vi "AlliGator Compute Optimal IRF v2.vi"(0 "Selected Plot Info":T8={"Multiplot XY Graph"=refnum, "Mouse Coordinates"={"Horizontal"=0, "Vertical"=0}, "Plot Index"=-1}, 5 "IRF*PSED Fixed Parameters":T3={"order"=0, "T"=0.0, "Time Constant Array"=[], "{S_k, C_k, phi_k, e_k} arrays"={"S_k Array"=[], "C_k Array"=[], "phi_k Array"=[], "e_k Array"=[]}, "IRF Extraction Options"={"Time Constant for IRF Extraction"=1e-18, "IRF Order"=0, "Fourier Series Smoothing"=enum."None", "Noise Threshold"=0.0, "Smoothing Width"=0.0, "Fourier Series Truncation"=enum."Automatic", "Truncation Order"=0, "Save Power Spectrum"=FALSE, "Smoothing"=FALSE, "Smoothing Parameter"=0.0, "Smoothing Order"=1, "Method"=enum."Direct"}} {"IRF Extraction Options"."Smoothing Order" min=1 max=10; "IRF Extraction Options"."Time Constant for IRF Extraction" format="%#_5g"}, 9 "IRF Optimization Control":T1={"Search Range"=1e-18, "Search Step"=1e-18, "Tail Threshold (%)"=1e-09, "Regularized IRF"=FALSE, "Export Plot"=FALSE, "Export Data"=FALSE, "Smooth Metrics"=FALSE, "S-G Side Points"=1, "S-G Polynomial Order"=3, "Metrics"=enum."Average"} {"S-G Polynomial Order" min=3 max=10; "S-G Side Points" min=1; "Tail Threshold (%)" min=0.0 max=100.0; "Search Range" min=0.0 max=1e-09}, 11 "Error In":errorcluster) -> (2 "Optimization Graph":cluster{"Ramp Pattern":dbl[], dbl[]}[](graph), 3 "Residuals Plot":cluster{"X Array":dbl[], "Y Array":dbl[]}, 4 "Fitted Plot":cluster{"X Array":dbl[], "Y Array":dbl[]}, 6 "Plot Name":string, 8 "Fit Parameter Values":dbl[](array[numeric]), 10 "Optimal Tau":dbl, 13 "Additional Data":variant, 14 "Fit Results String":string, 15 "Error Out":errorcluster)   [LabVIEW 2021, in "AlliGator IRF.lvlib"]
doc: "Extract IRF from provided decay using deconvolution and finding the minimal metrics."
uses:
  AlliGator IRF.lvlib
  <vilib>/Analysis/NI_AALBase.lvlib
  Settings/AlliGator Settings.lvlib
  Settings/AlliGator Settings List.ctl
  Time/Time.lvlib
  Fits/Fit Calculation Method.ctl
  Fits/Fits.lvlib
  Fits/Residual Type.ctl
  Fits/Decay Convolution/Decay Model.ctl
  Fits/Ramp Type.ctl
  <vilib>/Analysis/6fits.llb/Curve Fitting Criteria.ctl
  <vilib>/Analysis/NI_AALPro.lvlib
  Fits/Fit Settings.ctl
  Fits/D-Only Fixed Parameters.ctl
  Fits/Fit Models.ctl
  Fits/IRF(X)PSED/IRF(X)PSED Fit Parameters.ctl
  <vilib>/Utility/miscctls.llb/LVPointDoubleTypeDef.ctl
  Fits/Fit Plot Request Information.ctl
  Error/Error.lvlib
  Fits/Non-linear Fitting Algorithm.ctl
  Utilities/Utilities.lvlib
  Fits/IRF(X)PSED/Fourier Series Smoothing Option.ctl
  Fits/IRF(X)PSED/Fourier Series Truncation.ctl
  Fits/IRF(X)PSED/IRF(X)PSED Extraction Options.ctl
  Fits/IRF(X)PSED/IRF Extraction Method.ctl
  Fits/Non-linear Fitting Method v2.ctl
  Fits/Nonlinear Fit Method.ctl
  <vilib>/Analysis/1siggen.llb/Ramp Pattern by Delta.vi
  Fits/IRF(X)PSED/Fit Weights Type v2.ctl
  Fits/IRF(X)PSED/Decay Fit Options v4.ctl
  <vilib>/Utility/miscctls.llb/LVPoint32TypeDef.ctl
  Graphs/XY Graph/XY Graph Refnum.ctl
  Graphs/XY Graph/XY Graph Add-Ons.lvlib
  Graphs/XY Graph/XY Graph Selected Plot Info.ctl
  Fits/IRF(X)PSED/IRF(X)PSED Fixed Parameters v3.ctl
  AlliGator IRF Optimization Controls.ctl
  AlliGator IRF Deconvolution Metrics.ctl
panel:
  in  "Minimum Type":enum16{"Integral", "Chi 2", "Product"}(ring)=enum."Chi 2"
  out "Current Tau (ns)":dbl format="%#_4g"
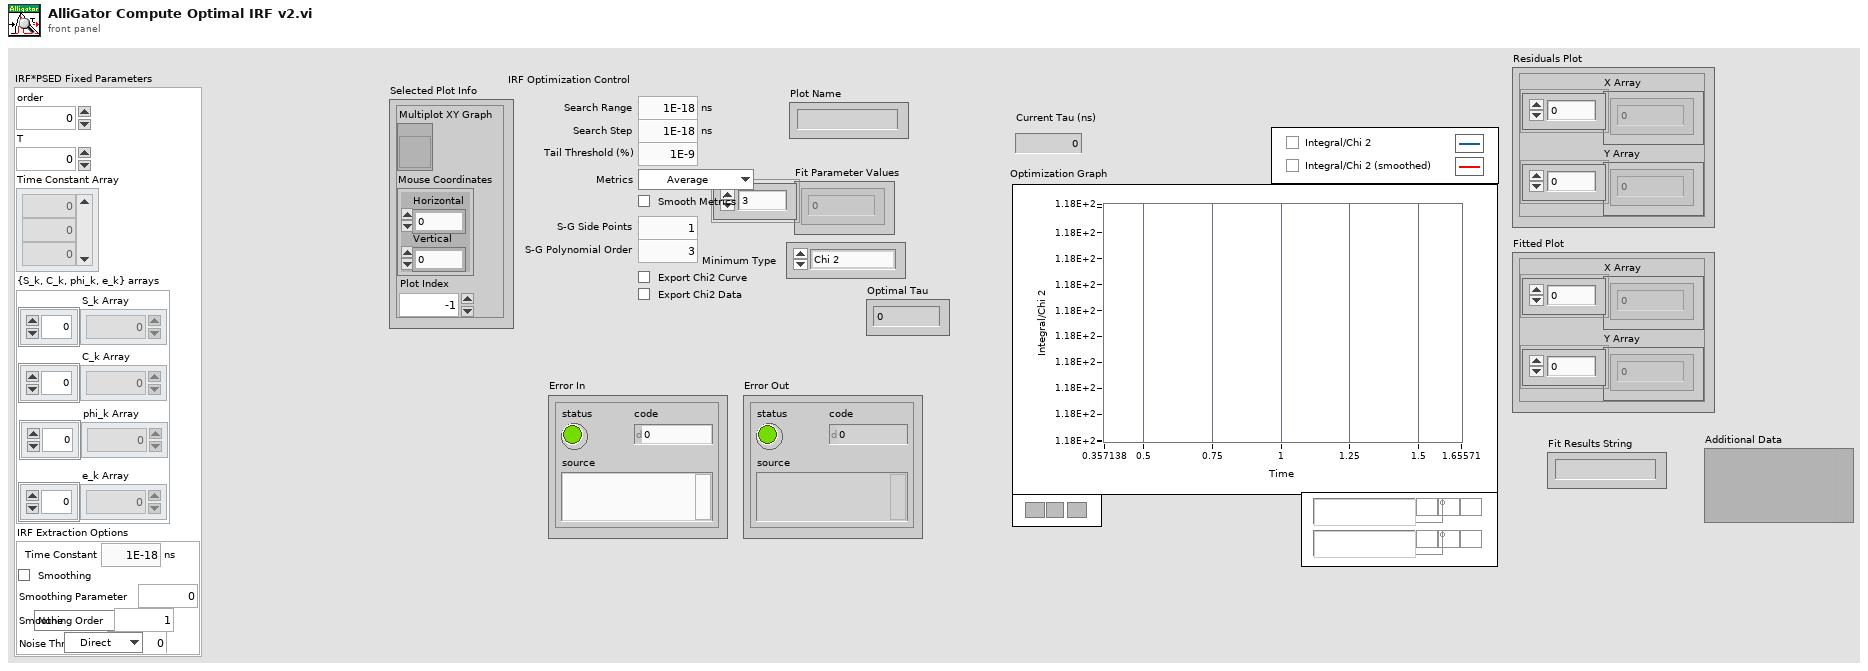
[diagram p1: front panel]
types:
  T1 = typedef "AlliGator IRF.lvlib/AlliGator IRF Optimization Controls.ctl" = cluster{"Search Range":dbl[unit], "Search Step":dbl[unit], "Tail Threshold (%)":dbl, "Regularized IRF":bool, "Export Plot":bool, "Export Data":bool, "Smooth Metrics":bool, "S-G Side Points":i32, "S-G Polynomial Order":i32, "Metrics":T2}
  T2 = typedef "AlliGator IRF.lvlib/AlliGator IRF Deconvolution Metrics.ctl" = enum16{"Average", "SDV", "Max", "Average * SDV", "Slope"}
  T3 = typedef "Fits.lvlib/IRF(X)PSED Fixed Parameters v3.ctl" = cluster{"order":i32, "T":dbl, "Time Constant Array":dbl[], "{S_k, C_k, phi_k, e_k} arrays":cluster{"S_k Array":dbl[], "C_k Array":dbl[], "phi_k Array":dbl[], "e_k Array":dbl[]}, "IRF Extraction Options":T4}
  T4 = typedef "Fits.lvlib/IRF(X)PSED Extraction Options.ctl" = cluster{"Time Constant for IRF Extraction":dbl[unit], "IRF Order":i32, "Fourier Series Smoothing":T5, "Noise Threshold":dbl, "Smoothing Width":dbl, "Fourier Series Truncation":T6, "Truncation Order":i32, "Save Power Spectrum":bool, "Smoothing":bool, "Smoothing Parameter":dbl, "Smoothing Order":u32, "Method":T7}
  T5 = typedef "Fits.lvlib/Fourier Series Smoothing Option.ctl" = enum16{"None", "Lanczos Factors", "Fejer Summation"}
  T6 = typedef "Fits.lvlib/Fourier Series Truncation.ctl" = enum16{"Automatic", "Fixed"}
  T7 = typedef "Fits.lvlib/IRF Extraction Method.ctl" = enum16{"Direct", "Topless", "Toeplitz"}
  T8 = typedef "XY Graph Add-Ons.lvlib/XY Graph Selected Plot Info.ctl" = cluster{"Multiplot XY Graph":T9, "Mouse Coordinates":T10, "Plot Index":i32}
  T9 = typedef "XY Graph Add-Ons.lvlib/XY Graph Refnum.ctl" = refnum<vi>
  T10 = typedef "LVPoint32TypeDef.ctl" = cluster{"Horizontal":i32, "Vertical":i32}
  T11 = typedef "Fits.lvlib/Fit Settings.ctl" = cluster{"Use Original Plot # Points":bool, "# Fit Plot Points":u32, "Fitting Method":T12, "Weighted Fit":T13, "Show All Fit Components":bool, "Axis Type":T14, "Show Fit Residuals":bool, "Residual Type":T15, "Fitting Algorithm":T16, "Show Confidence Interval":bool, "Confidence Level":dbl}
  T12 = typedef "Fits.lvlib/Nonlinear Fit Method.ctl" = enum16{"Least Square", "Least Absolute Residual", "Bisquare", "MLE"}
  T13 = typedef "Fits.lvlib/Fit Weights Type v2.ctl" = enum16{"Unweighted", "1/Variance (Neyman)", "1/Variance (Pearson)", "Best of All"}
  T14 = typedef "Fits.lvlib/Ramp Type.ctl" = u16
  T15 = typedef "Fits.lvlib/Residual Type.ctl" = enum16{"Standard", "Normalized", "Reduced"}
  T16 = typedef "Fits.lvlib/Non-linear Fitting Algorithm.ctl" = enum16{"Levenberg-Marquardt", "Trust-Region Dogleg"}
  T17 = typedef "Fits.lvlib/Decay Fit Options v4.ctl" = cluster{"Show Fit Residuals":bool, "Fit Model":T18, "Residual Type":T15, "Max Decay Percentile":dbl, "Min Decay Percentile":dbl, "Show Full Decay":bool, "Weights":T13, "Fitting Method":T19, "Compute Parameter Uncertainties":bool, "Periodic Boundaries":bool, "Model Calculation":T20, "Period":dbl[unit], "Termination Criteria":cluster{"Max Iterations":i32, "Max Function Calls":i32, "Max Time":dbl[unit], "Function Tolerance":dbl, "Parameter Tolerance":dbl, "Gradient Tolerance":dbl, "Min Lambda":dbl, "Max Lambda":dbl, "Initial Tick Count":u32}, "Offset Resolution":dbl[unit], "Use Local IRF":bool, "Fitting Algorithm":T16, "Show Confidence Interval ":bool, "Confidence Level":dbl}
  T18 = typedef "Fits.lvlib/Decay Model.ctl" = enum16{"1-Exponential", "2-Exponentials"}
  T19 = typedef "Fits.lvlib/Non-linear Fitting Method v2.ctl" = enum16{"Least Square", "Least Absolute Residual", "Bisquare", "MLE", "-", "Best of All"}
  T20 = typedef "Fits.lvlib/Fit Calculation Method.ctl" = enum16{"Simulation", "Convolution", "Integration"}
  T21 = typedef "AlliGator Settings.lvlib/AlliGator Settings List.ctl" = enum16{"GUI:Visible Settings Tab", "GUI:Last Run Version", "Source Image:Use Image Histogram for Contrast", "Source Image:Low Count Pixels Rejection Options", "Source Image:High Count Pixels Rejection Options", "Source Image:Use Image Brightness", "Source Image:Blend Overlay with Image Background", "Source Image:Use Fixed ROI Diameter", "Source Image:ROI Diameter", "Source Image:ROI Center Color", "Source Image:Peak Threshold", "Source Image:Intensity Threshold", "Source Image:Image Binning Options", "Source Image:Image Smoothing Options", "Source Image:Image Histogram Active", "Source Image:Invert Binary Mask", "Source Image:Hot Pixel Removal", "Source Image:Overlay Analyzed ROI Center", "Source Image:Auto-Adjust Contrast", "Source Image:Histogram Lower Percentile", "Source Image:Histogram Upper Percentile", "Source Image:Save Source Image", "Source Image:Scale Bar Options", "Source Image:Image Resolution (Pixel Size)", "Source Image:Flatfield Correction", "Source Image:Show Dead Left Columns Correction", "Source Image:Dead Left Columns Correction", "Source Image:Image Pre-Processing Operations Order", "Source Image:Overlay ROI Median", "Source Image:Median Overlay Color", "Data Information:Gate Width", "Data Information:Nanotime Gate Separation", "Data Information:Macrotime Gate Separation", "Data Information:Gate Step", "Data Information:# Gates", "Data Information:Gate Image Exposure", "Data Information:Gate Image Integration", "Data Information:Gates to Skip", "Data Information:Gates to Keep", "Data Information:Define Gates to", "Data Information:Channel Name", "Data Information:Available Channel Names", "Data Information:Channel Arithmetic", "Data Information:Background File Subtraction", "Data Information:Background File", "Data Information:Background Scaling Factor", "Data Information:Background Pile-up Correction", "Data Information:Background Pixel Well Capacity", "Data Information:Laser Period", "Data Information:SYNC Period", "Data Information:Pile-up Correction", "Data Information:Pixel Well Capacity", "Data Information:Dataset Scaling Factor", "Fluorescence Decay_Decay Pre-Processing:Reverse Gates", "Fluorescence Decay_Decay Pre-Processing:Verbose Decay Pre-Processing", "Fluorescence Decay_Decay Pre-Processing:Use Decay Pre-Processing", "Fluorescence Decay_Decay Pre-Processing:Background Subtraction", "Fluorescence Decay_Decay Pre-Processing:Background Definition Range", "Fluorescence Decay_Decay Pre-Processing:Baseline Subtraction Method", "Fluorescence Decay_Decay Pre-Processing:Decay Pre-Processing Operations Order", "Fluorescence Decay_Decay Pre-Processing:Smoothing Parameter", "Fluorescence Decay_Decay Pre-Processing:Shift Decay", "Fluorescence Decay_Decay Pre-Processing:Decay Shift Parameters", "Fluorescence Decay_Decay Pre-Processing:Fold Decay", "Fluorescence Decay_Decay Pre-Processing:# Folds", "Fluorescence Decay_Decay Pre-Processing:1-Normalize Decay", "Fluorescence Decay_Decay Pre-Processing:[0-1]-Normalize Decay", "Fluorescence Decay_Decay Pre-Processing:Smoothen Decay", "Fluorescence Decay_Decay Pre-Processing:Extrapolate Decay", "Fluorescence Decay_Decay Pre-Processing:Use Periodicity", "Fluorescence Decay_Decay Pre-Processing:Use Cursors", "Fluorescence Decay_Decay Pre-Processing:Tail Fraction", "Fluorescence Decay_Decay Pre-Processing:Head Fraction", "Fluorescence Decay_Decay Pre-Processing:Additional Points", "Fluorescence Decay_Decay Pre-Processing:Straighten Decay", "Fluorescence Decay_Decay Pre-Processing:Constant Background", "Fluorescence Decay_Decay Pre-Processing:Pixel-Normalize Decay", "Fluorescence Decay_Advanced Analysis:Extract IRF instead of Decay", "Fluorescence Decay_Advanced Analysis:IRF Extraction Options", "Fluorescence Decay_Advanced Analysis:IRF Optimization Options", "Fluorescence Decay_Advanced Analysis:Square Pulse Options", "Fluorescence Decay_Advanced Analysis:IRF Order", "Fluorescence Decay_Advanced Analysis:IRF Time Constants", "Fluorescence Decay_Advanced Analysis:Wavelet Analysis Options", "Fluorescence Decay_Advanced Analysis:Average Lifetime Options", "Fluorescence Decay_Fit Options:Fit Options", "Fluorescence Decay_Fit Options:Use Legacy Fitting Approach", "Fluorescence Decay_Fit Options:Use Data Information Laser Period", "Fluorescence Decay_Fit Parameters:Displayed Fit Parameters", "Fluorescence Decay_Fit Parameters:Fit Parameter Constraints", "Fluorescence Decay_Fit Parameters:Export Tabulated Results", "Fluorescence Decay_Fit Parameters:MLE Baseline Offset Type", "Fluorescence Decay_Fit Parameters:MLE Baseline Offset", "Fluorescence Decay_Fit Parameters:Guess Parameter Names", "Fluorescence Decay_Fit Parameters:Guess Parameter Values", "Fluorescence Decay_Fit Parameters:Guess Parameters Options", "Fluorescence Decay_Fit Parameters:Optimal Offset Selection Criterion", "Fluorescence Decay_Styles:Show Last Decay Only", "Fluorescence Decay_Styles:Decay Graph Color Array", "Fluorescence Decay:Decay Graph Active", "Fluorescence Decay Statistics:Min Peak Value", "Fluorescence Decay Statistics:Reject Low Decay Peak Pixels", "Fluorescence Decay Statistics:Reject High Decay Peak Pixels", "Fluorescence Decay Statistics:Max Peak Value", "Time Traces:Use File Timestamp", "Time Traces:Time Step", "Time Traces:Use Intensity Correction File", "Time Traces:Intensity Correction File", "Phasor Plot:Phasor Plot Smoothing Options", "Phasor Plot:Phasor Plot Size", "Phasor Plot:Phasor Plot Graphics Options", "Phasor Plot:Cumulative Phasor Plot", "Phasor Plot:Use Phasor Brightness", "Phasor Plot:Blend Overlay with Phasor Background", "Phasor Plot:Save Phasor Plot", "Phasor Plot:Show References", "Phasor Plot:Phasor Ratio Decay Range", "Phasor Plot:Exponential Fading", "Phasor Plot:Phasor Ratio Reference Colors", "Phasor Plot:Reference Radius", "Phasor Plot:Show Color Map Vertices", "Phasor Plot:Phasor Plot Active", "Phasor Plot:Phasor Ratio Color Map Type", "Phasor Plot:Phasor Ratio Color Map", "Phasor Plot:Phasor Ratio Display Range", "Phasor Plot:Selected Image ROI(s)", "Phasor Plot:All Image ROIs", "Phasor Plot:Selected Phasor Plot ROI(s)", "Phasor Plot:All Phasor Plot ROIs", "Phasor Plot:Phasor Ratio Color-Coded Quantity", "Phasor Plot:Store Phasor Harmonics", "Phasor Plot:Draw Reference Segment", "Phasor Plot:User-Defined Quantity", "Phasor Plot:Color Scale High Color", "Phasor Plot:Color Scale Low Color", "Phasor Plot:Intensity-weighted Phasor Plot", "Phasor Graph:Phasor Frequency", "Phasor Graph:Phasor Ratio Type", "Phasor Graph:Pixel-level Phasor Computation", "Phasor Graph:Save Phasor Graph", "Phasor Graph:Phasor Graph Active", "Phasor Graph:Phasor SDV Options", "Phasor Graph:Intensity-weighted Phasor Graph", "Phasor Graph:Define Shortest Lifetime as", "Phasor Calibration:Use Backup Calibration if needed", "Phasor Calibration:Backup Calibration Type", "Phasor Calibration:Calibration Type", "Phasor Calibration:Calibration Lifetime", "Phasor Calibration:Calibration Map Algorithm", "Single-Exponential Phasor Locus (SEPL):Gate Parameters", "Single-Exponential Phasor Locus (SEPL):User-defined Gate", "Single-Exponential Phasor Locus (SEPL):User-defined IRF", "Single-Exponential Phasor Locus (SEPL):Phasor Parameters", "Single-Exponential Phasor Locus (SEPL):Decay & IRF Parameters", "Single-Exponential Phasor Locus (SEPL):Display Parameters", "Lifetime Analysis:Decay Analysis Parameters", "Lifetime Analysis:Lifetime Map Active", "Plugins:Python Settings", "Miscellaneous:Verbose Mode", "Miscellaneous:Beep after Script", "Miscellaneous:Saved Image File Format", "Miscellaneous:Exported Gate Image Settings", "Miscellaneous:Include Loading in Timing", "Miscellaneous:Verbose Settings Mode", "Miscellaneous:Histogram Options", "Miscellaneous:Beep on Error", "Miscellaneous:# Logical Processors Used", "Miscellaneous:ROI Description Max Characters", "Miscellaneous:Verbose Error Mode", "Miscellaneous:Transparent Mask Color"}
  T22 = typedef "Fits.lvlib/Fit Plot Request Information.ctl" = cluster{"XY Graph Ref":refnum<vi>, "Mouse Coordinates":T23, "Fit Model":T24, "Plot Index":i32}
  T23 = typedef "LVPointDoubleTypeDef.ctl" = cluster{"X":dbl, "Y":dbl}
  T24 = typedef "Fits.lvlib/Fit Models.ctl" = enum16{"Select a Fit Model...", "           Single Peak", "Gaussian", "Asymmetric Gaussian", "Lorentzian", "Asymmetric Lorentzian", "Gaussian/Lorentzian", "Lorentzian/Gaussian", "           Double Peak", "Two Gaussians", "Two Asymmetric Gaussians", "Two H-Connected Gaussians", "Two T-Connected Gaussians", "Two H-Connected Asymmetric Gaussians", "Two T-Connected Asymmetric Gaussians", "           Triple Peak", "Three Gaussians", "Three Asymmetric Gaussians", "              Decays", "1-Exponential", "IRF*PSED", "2-Exponentials", "            Power Law", "Power Law", "Power Law with Offset", "               ACF", "2D Gaussian ACF", "2D Gaussian + Blinking ACF", "2D Gaussian + Flow ACF", "3D Gaussian ACF", "3D Gaussian + Blinking ACF", "             Multiplot", "2D Gaussian ACF & 2D Gaussian + Flow ACF"}
  T25 = typedef "Fits.lvlib/IRF(X)PSED Fit Parameters.ctl" = cluster{"Offset":dbl, "Amplitudes":dbl[], "Time Constants":dbl[], "Baseline":dbl, "Lifetime":dbl, "IRF order":dbl, "Period":dbl, "SDV":dbl, "FWHM":dbl, "Integral":dbl, "MSE":dbl, "R^2":dbl}
  T26 = typedef "Fits.lvlib/D-Only Fixed Parameters.ctl" = cluster{"Fix D-only Peak Location":bool, "Peak Location":dbl, "Fix D-only Peak FWHM":bool, "Peak FWHM":dbl}
  T27 = typedef "NI_AALPro.lvlib/Curve Fitting Criteria.ctl" = u16
  T28 = typedef "Fits.lvlib/Fit Model Information.ctl" = cluster{"Fit Model":T24, "LM Function & Gradient":refnum<vi>, "Additional Fit Settings":variant}
  T29 = typedef "Fits.lvlib/Fit Output Data.ctl" = cluster{"Fit Parameters Cluster":variant, "Fit Parameters Uncertainties Cluster":variant, "Additional Data":variant}
  T30 = cluster{"Ramp Pattern":dbl[], "Best Polynomial Fit":dbl[]}
  T31 = cluster{"Ramp Pattern":dbl[], "Best Polynomial Fit":dbl[]}[]
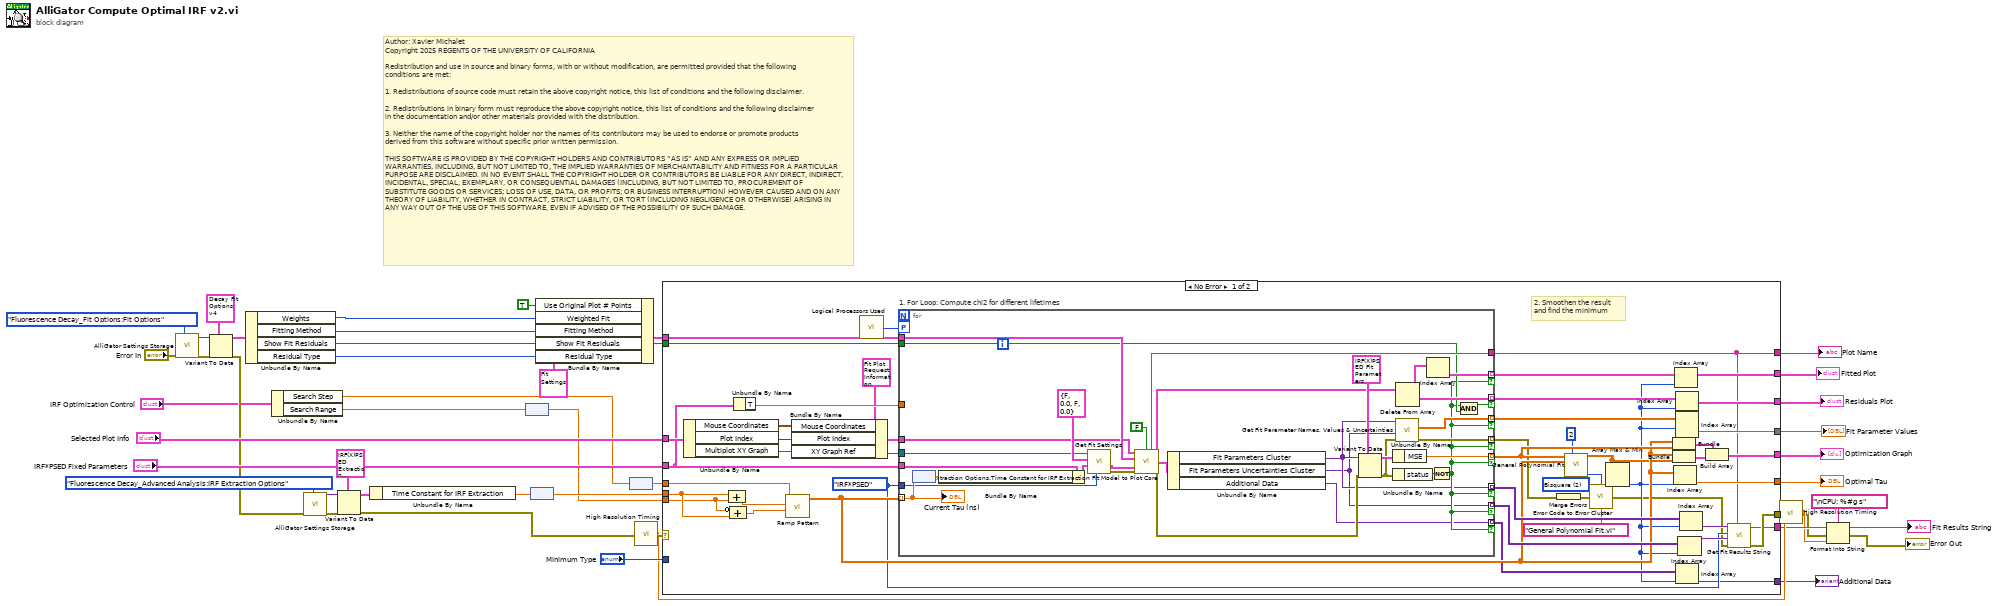
[diagram p0: block diagram]
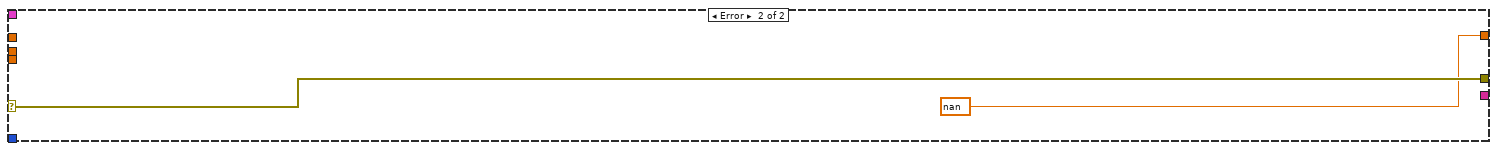
[diagram p2: hidden frame]
diagram:
  # "Author: Xavier Michalet\nCopyright 2025 REGENTS OF THE UNIVERSITY OF CALIFORNIA\n\nRedistribution and use in source and binary forms, with or without modification, are permitted provided that the following conditions are met:\n\n1. Redistributions of source code must retain the above copyright notice, this list of conditions and the following disclaimer.\n\n2. Redistributions in binary form must reproduce the above copyright notice, this list of conditions and the following disclaimer in the documentation and/or other materials provided with the distribution.\n\n3. Neither the name of the copyright holder nor the names of its contributors may be used to endorse or promote products derived from this software without specific prior written permission.\n\nTHIS SOFTWARE IS PROVIDED BY THE COPYRIGHT HOLDERS AND CONTRIBUTORS “AS IS” AND ANY EXPRESS OR IMPLIED WARRANTIES, INCLUDING, BUT NOT LIMITED TO, THE IMPLIED WARRANTIES OF MERCHANTABILITY AND FITNESS FOR A PARTICULAR PURPOSE ARE DISCLAIMED. IN NO EVENT SHALL THE COPYRIGHT HOLDER OR CONTRIBUTORS BE LIABLE FOR ANY DIRECT, INDIRECT, INCIDENTAL, SPECIAL, EXEMPLARY, OR CONSEQUENTIAL DAMAGES (INCLUDING, BUT NOT LIMITED TO, PROCUREMENT OF SUBSTITUTE GOODS OR SERVICES; LOSS OF USE, DATA, OR PROFITS; OR BUSINESS INTERRUPTION) HOWEVER CAUSED AND ON ANY THEORY OF LIABILITY, WHETHER IN CONTRACT, STRICT LIABILITY, OR TORT (INCLUDING NEGLIGENCE OR OTHERWISE) ARISING IN ANY WAY OUT OF THE USE OF THIS SOFTWARE, EVEN IF ADVISED OF THE POSSIBILITY OF SUCH DAMAGE."
  n1 = call "AlliGator Settings Storage.vi"("AlliGator Settings List"=AlliGator_Settings_List."Fluorescence Decay_Fit Options:Fit Options", "Error In"="Error In") -> ("Error Out"=w34:errorcluster, "Variant Data out"=w33:variant)  [unwired: 8 in]
  n2 = Variant To Data(error in=w34, type=T17 {"Show Fit Residuals"=TRUE, "Fit Model"=enum."1-Exponential", "Residual Type"=enum."Standard", "Max Decay Percentile"=0.0, "Min Decay Percentile"=0.0, "Show Full Decay"=TRUE, "Weights"=enum."Unweighted", "Fitting Method"=enum."Least Square", "Compute Parameter Uncertainties"=TRUE, "Periodic Boundaries"=TRUE, "Model Calculation"=enum."Simulation", "Period"=1.2500000000000001e-08, "Termination Criteria"={"Max Iterations"=1000, "Max Function Calls"=0, "Max Time"=1000.0, "Function Tolerance"=1e-06, "Parameter Tolerance"=1e-06, "Gradient Tolerance"=0.0, "Min Lambda"=1e-06, "Max Lambda"=1e-06, "Initial Tick Count"=0}, "Offset Resolution"=1.2500000000000001e-08, "Use Local IRF"=TRUE, "Fitting Algorithm"=enum."Levenberg-Marquardt", "Show Confidence Interval "=TRUE, "Confidence Level"=95.0} ("Fit Options"), Variant=w33) -> (data=w31:T17, error out=w25:errorcluster)
  n3 = Unbundle By Name(w31) -> ("Weights"=w1:T13, "Fitting Method"=w29:T19, "Show Fit Residuals"=w15:bool, "Residual Type"=w28:T15)
  n4 = Unbundle By Name("IRF Optimization Control") -> ("Search Step"=w4:dbl[unit], "Search Range"=w3:dbl[unit])
  n5 = call "AlliGator Settings Storage.vi"("AlliGator Settings List"=AlliGator_Settings_List."Fluorescence Decay_Advanced Analysis:IRF Extraction Options", "Error In"=w25) -> ("Error Out"=w24:errorcluster, "Variant Data out"=w44:variant)  [unwired: 8 in]
  n6 = Variant To Data(error in=w24, type=T4 {"Time Constant for IRF Extraction"=1e-18, "IRF Order"=1, "Fourier Series Smoothing"=enum."None", "Noise Threshold"=0.0, "Smoothing Width"=0.0, "Fourier Series Truncation"=enum."Automatic", "Truncation Order"=0, "Save Power Spectrum"=FALSE, "Smoothing"=FALSE, "Smoothing Parameter"=0.0, "Smoothing Order"=1, "Method"=enum."Direct"} ("IRF Extraction Options"), Variant=w44) -> (data=w45:T4, error out=w23:errorcluster)
  n7 = Unbundle By Name(w45) -> ("Time Constant for IRF Extraction"=w6:dbl[unit])
  n8 = node(w3) -> (w2:dbl)
  n9 = node(w6) -> (w38:dbl)
  n10 = Bundle By Name(cluster=T11 {"Use Original Plot # Points"=TRUE, "# Fit Plot Points"=0, "Fitting Method"=enum."Least Square", "Weighted Fit"=enum."Unweighted", "Show All Fit Components"=FALSE, "Axis Type"=0, "Show Fit Residuals"=FALSE, "Residual Type"=enum."Standard", "Fitting Algorithm"=enum."Levenberg-Marquardt", "Show Confidence Interval"=TRUE, "Confidence Level"=95.0} ("Fit Settings"), "Use Original Plot # Points"=TRUE, "Weighted Fit"=w1, "Fitting Method"=w29, "Show Fit Residuals"=w15, "Residual Type"=w28) -> (w27:T11)
  n11 = node(w4) -> (w39:dbl)
  n12 = call "High Resolution Timing.vi"("Error In"=w23) -> ("elapsed (relative) seconds"=w22:dbl, "Error Out"=w41:errorcluster)  [unwired: 16 in, 1 out]
  n13 = case shown="No Error" w41 {
    selector: w41 -> [_ w127]
    tunnel: [w64 w127] -> w46
    tunnel: w38 -> [w91 _]
    tunnel: [w83 nan] -> w42
    tunnel: "Minimum Type" -> [_ _]
    tunnel: w39 -> [w90 _]
    tunnel: w2 -> [w89 _]
    tunnel: "Selected Plot Info" -> [w86 _]
    tunnel: "IRF*PSED Fixed Parameters" -> [w85 _]
    tunnel: w27 -> [w87 _]
    tunnel: [w77 _] -> w21
    tunnel: [w63 _] -> w20
    tunnel: [w75 _] -> w19
    tunnel: [w73 _] -> w18
    tunnel: [w71 _] -> w16
    tunnel: w15 -> [w70 _]
    tunnel: [w62 _] -> w14
    tunnel: [w52 _] -> w8
    frame No Error {
      w59 = T27 2 items=["Least Square", "Least Absolute Residual", "Bisquare"] ("method")
      w55 = Fit_Models."IRF*PSED" ("Fit Model")
      # "2. Smoothen the result\nand find the minimum"
      n14 = Unbundle By Name(w86) -> ("Mouse Coordinates"=w79:T10, "Plot Index"=w78:i32, "Multiplot XY Graph"=w80:T9)
      n15 = Compound Arithmetic op=ADD(w91, w89) -> (w93:dbl)
      n16 = Compound Arithmetic op=ADD(invert w89, w91) -> (w92:dbl)
      n17 = Unbundle By Name(w85) -> ("T"=w84:dbl)
      n18 = call-poly <vilib>:"Ramp Pattern.vi"("start"=w92, "end"=w93, "delta"=w90) -> ("Ramp Pattern"=w60:dbl[])  [unwired: 6 in, 2 out]
      n19 = Bundle By Name(cluster=T22 {"XY Graph Ref"=refnum, "Mouse Coordinates"={"X"=0.0, "Y"=0.0}, "Fit Model"=enum."IRF*PSED", "Plot Index"=-1} ("Fit Plot Information"), "Mouse Coordinates"=w79, "Plot Index"=w78, "XY Graph Ref"=w80) -> (w81:T22)
      n20 = call "Logical Processors Used.vi"() -> ("# Logical Processor Used"=w51:i32)  [unwired: 6 in]
      n21 = for "1. For Loop: Compute chi2 for different lifetimes" {
        tunnel: w60 -> [w124] mode=indexing
        workers-P: w51 -> [_]
        tunnel: w87 -> [w120]
        tunnel: w85 -> [w125]
        tunnel: w80 -> [w113]
        tunnel: [w115] -> w61 mode=indexing if=w99
        tunnel: w84 -> [_]
        tunnel: w81 -> [w112]
        tunnel: [w111] -> w63
        tunnel: [w110] -> w76 mode=indexing if=w99
        tunnel: [w109] -> w49 mode=indexing if=w99
        tunnel: [w107] -> w74 mode=indexing if=w103
        tunnel: [w104] -> w72 mode=indexing if=w99
        tunnel: w70 -> [w102]
        tunnel: [w96] -> w68 mode=indexing if=w99
        tunnel: [w95] -> w67 mode=indexing if=w99
        tunnel: w55 -> [w101]
        tunnel: [w94] -> w54 mode=indexing if=w99
        n22 = node(w124) -> (w98:dbl[unit])
        n23 = Bundle By Name(cluster=w125, "IRF Extraction Options.Time Constant for IRF Extraction"=w98) -> (w123:T3)
        n24 = call "Get Fit Settings.vi"("Fit Model"=w101, "Additional Parameters"=w123, "Fixed Parameters"=T26 {"Fix D-only Peak Location"=FALSE, "Peak Location"=0.0, "Fix D-only Peak FWHM"=FALSE, "Peak FWHM"=0.0}, "XY Graph Ref"=w113) -> ("Error Out"=w121:errorcluster, "Fit Model Information"=w97:T28)  [unwired: 4 in, 2 out]
        n25 = call "Fit Model to Plot Core.vi"("Fit Plot Information"=w112, "Display Plots (T)"=FALSE, "Fit Settings"=w120, "Fit Model Information"=w97, "error in (no error)"=w121) -> ("Plot Name"=w111:string, "Array of Plots (Fit, Components, Residuals)"=w106:cluster{"X Array":dbl[], "Y Array":dbl[]}[], "Fit Output Data"=w100:T29, "error out"=w117:errorcluster)  [unwired: 5 in, 2 out]
        n26 = Unbundle By Name(w100) -> ("Fit Parameters Cluster"=w96:variant, "Fit Parameters Uncertainties Cluster"=w95:variant, "Additional Data"=w94:variant)
        n27 = Variant To Data(error in=w117, type=T25 {"Offset"=0.0, "Amplitudes"=[], "Time Constants"=[], "Baseline"=0.0, "Lifetime"=0.0, "IRF order"=0.0, "Period"=0.0, "SDV"=0.0, "FWHM"=0.0, "Integral"=0.0, "MSE"=0.0, "R^2"=0.0} ("IRF*PSED Fit Parameters"), Variant=w96) -> (data=w118:T25, error out=w114:errorcluster)
        n28 = Unbundle By Name(w118) -> ("MSE"=w115:dbl)
        n29 = Unbundle By Name(w114) -> ("status"=w116:bool)
        n30 = call "Get Fit Parameter Names, Values & Uncertainties.vi"("error in (no error)"=w114, "Fit Parameter Uncertainties"=w95, "Fit Parameters"=w96) -> ("Error Out"=w109:errorcluster, "Fit Parameter Values"=w110:dbl[])  [unwired: 5 in, 2 out]
        n31 = Delete From Array(array=w106) -> (deleted portion=w107:cluster{"X Array":dbl[], "Y Array":dbl[]}, array with subset deleted=w105:cluster{"X Array":dbl[], "Y Array":dbl[]}[])  [unwired: 2 in]
        n32 = Index Array(array=w105) -> (element=w104:cluster{"X Array":dbl[], "Y Array":dbl[]})  [unwired: 1 in]
        n33 = Not(x=w116) -> (.not. x?=w99:bool)
        n34 = Compound Arithmetic op=AND(w99, w102) -> (w103:bool)
        "Current Tau (ns)" <- w124
      }
      n35 = Merge Errors(w49) -> (w48:errorcluster)
      n36 = call <vilib>:"General Polynomial Fit.vi"("Y"=w61, "polynomial order"=2, "X"=w60, "method"=w59) -> ("Best Polynomial Fit"=w57:dbl[], "error"=w56:i32)  [unwired: 8 in, 2 out]
      n37 = call "Error Code to Error Cluster.vi"("Error Code"=w56, "Error Source"="General Polynomial Fit.vi", "Error In"=w48) -> ("Error Out"=w50:errorcluster)  [unwired: 12 in]
      n38 = Array Max & Min(array=w57) -> (min index (indices)=w53:i32)  [unwired: 3 out]
      n39 = Bundle("Ramp Pattern"=w60, w61) -> (w69:cluster{"Ramp Pattern":dbl[], dbl[]})  [unwired: 1 in]
      n40 = Bundle("Ramp Pattern"=w60, "Best Polynomial Fit"=w57) -> (w88:T30)  [unwired: 1 in]
      n41 = Index Array(array=w60, index=w53) -> (element=w83:dbl)
      n42 = Index Array(array=w72, index=w53) -> (element=w71:cluster{"X Array":dbl[], "Y Array":dbl[]})
      n43 = Index Array(array=w74, index=w53) -> (element=w73:cluster{"X Array":dbl[], "Y Array":dbl[]})
      n44 = Index Array(array=w76, index (row)=w53) -> (element=w75:dbl[])  [unwired: 1 in]
      n45 = Index Array(array=w54, index=w53) -> (element=w52:variant)
      n46 = Index Array(array=w67, index=w53) -> (element=w65:variant)
      n47 = Index Array(array=w68, index=w53) -> (element=w66:variant)
      n48 = Build Array(w69, w88) -> (w77:T31)
      n49 = call "Get Fit Results String.vi"("Plot Name"=w63, "error in (no error)"=w50, "Fit Parameters Uncertainties Cluster"=w65, "Fit Model"=w55, "Fit Parameters Cluster"=w66) -> ("error out"=w64:errorcluster, "Fit Results String"=w62:string)  [unwired: 5 in]
    }
    frame Error {
    }
  }
  "Optimal Tau" <- w42
  "Optimization Graph" <- w21
  "Plot Name" <- w20
  "Fit Parameter Values" <- w19
  "Residuals Plot" <- w18
  "Fitted Plot" <- w16
  "Additional Data" <- w8
  n50 = call "High Resolution Timing.vi"("relative seconds (NaN)"=w22, "Error In"=w46) -> ("elapsed (relative) seconds"=w12:dbl, "Error Out"=w10:errorcluster)  [unwired: 15 in, 1 out]
  n51 = Format Into String(format string="\nCPU: %#g s", initial string=w14, error in=w10, w12) -> (resulting string=→"Fit Results String":string, error out=→"Error Out":errorcluster)
